vi "Destroy.vi"(8 "error in (no error)":errorcluster, 11 "XRay Cabinet in":refnum<class "XRay Cabinet.lvclass">) -> (0 "error out":errorcluster, 3 "XRay Cabinet out":refnum<class "XRay Cabinet.lvclass">)   [LabVIEW 2026, in "XRay Cabinet.lvclass"]
uses:
  XRay Cabinet.lvclass
  XRay Cabinet.lvclass/XRay Cabinet.ctl
  XRay Scene/XRay Scene.lvclass
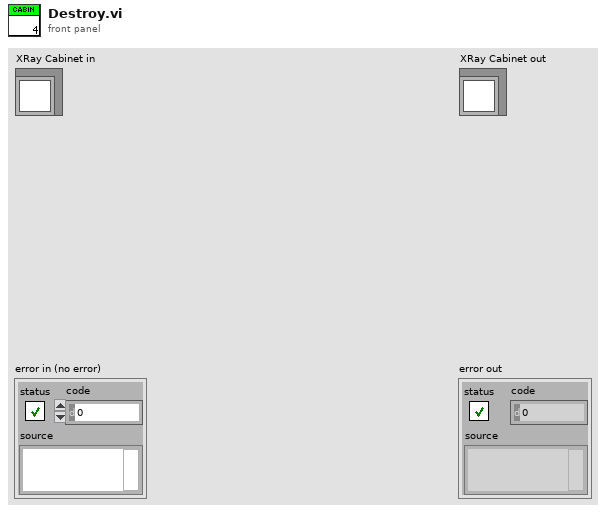
[diagram p1: front panel]
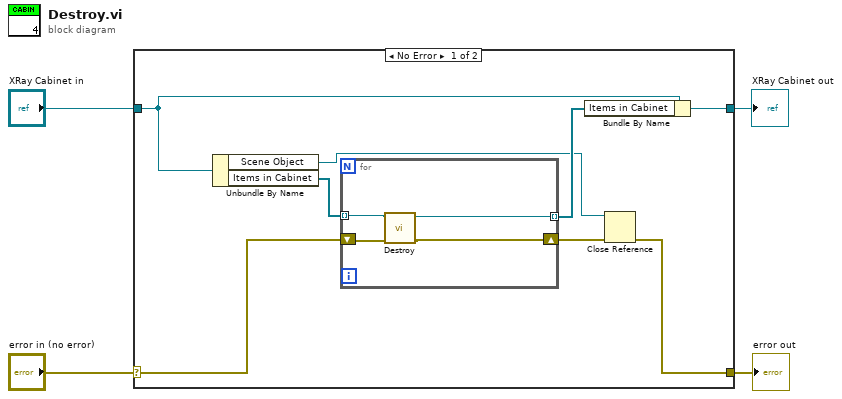
[diagram p0: block diagram]
diagram:
  n1 = case shown="No Error" "error in (no error)" {
    selector: "error in (no error)" -> [w8 w18]
    tunnel: [w6 w18] -> w3
    tunnel: [w9 w17] -> w1
    tunnel: "XRay Cabinet in" -> [w10 w17]
    frame No Error {
      n2 = Unbundle By Name(w10) -> ("Scene Object"=w5:refnum<vi>, "Items in Cabinet"=w11:refnum<class "XRay Scene.lvclass">[])
      n3 = for {
        tunnel: w11 -> [w16] mode=indexing
        tunnel: [w15] -> w12 mode=indexing
        shift-right: [w14] -> w7
        shift-left: w8 -> [w13]
        n4 = call-dynamic "Destroy.vi"("error in (no error)"=w13, "XRay Scene in"=w16) -> ("error out"=w14:errorcluster, "XRay Scene out"=w15:refnum<class "XRay Scene.lvclass">)  [unwired: 8 in]
      }
      n5 = Bundle By Name(cluster=w10, "Items in Cabinet"=w12) -> (w9:refnum<class "XRay Cabinet.lvclass">)
      n6 = Close Reference(reference=w5, error in (no error)=w7) -> (error out=w6:errorcluster)
    }
    frame Error {
    }
  }
  "error out" <- w3
  "XRay Cabinet out" <- w1
